vi "Mock Call Template VI.vi"(8 "error in (no error)":errorcluster, 11 "Mock In":refnum<class "LMock Mock.lvclass">) -> (3 "Mock Out":refnum<class "LMock Mock.lvclass">)   [LabVIEW 2020, in "Templates.lvlib"]
uses:
  Templates.lvlib
  Framework/Mock/LMock Mock.lvclass
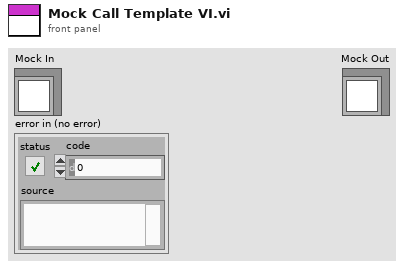
[diagram p1: front panel]
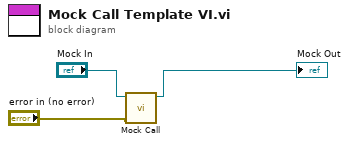
[diagram p0: block diagram]
diagram:
  n1 = call "Mock Call.vi"("error in (no error)"="error in (no error)", "Mock In"="Mock In") -> ("Mock Out"=→"Mock Out":refnum<class "LMock Mock.lvclass">)  [unwired: 8 in, 1 out]
